vi "tipos.vi"() -> ()   [LabVIEW 2013]
panel:
  out "Boolean Indicator/Output":bool
  in  "Boolean Control/Input":bool
  in  "Stop Button":bool
  out "Double-precision, floating-point Indicator/Output":dbl
  in  "Byte unsigned integer 0 to 255  Control/Input":u8
  out "Horizontal Graduated Bar Indicator/Output":u8(slide) scale=0.0..100.0
  in  "Vertical Pointer Slide Input Control/Input":dbl(slide) scale=0.0..10.0
  out "Gauge Indicator/Output":dbl(knob) scale=0.0..10.0
  out "String Indicator/Output":string
  in  "String Control/Input":string
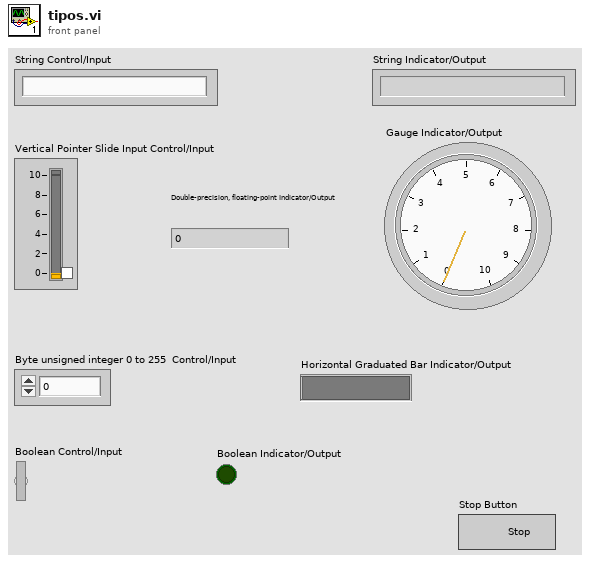
[diagram p1: front panel]
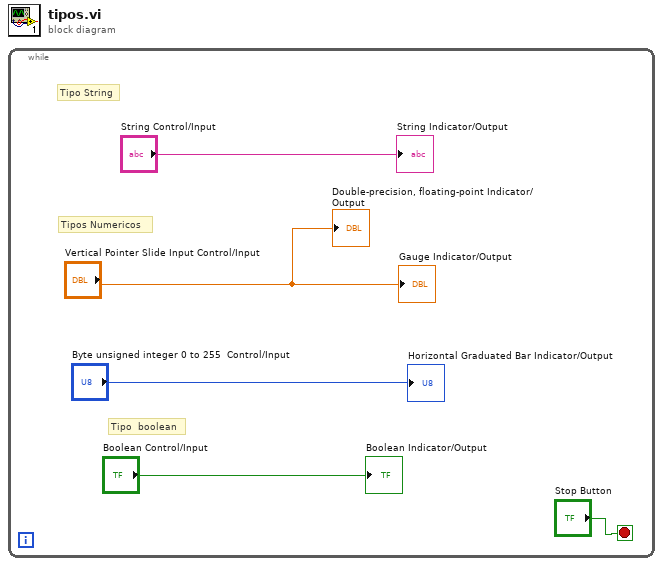
[diagram p0: block diagram]
diagram:
  n1 = while {
    stop <- "Stop Button" stop-if-true
    # "Tipo  boolean"
    # "Tipo String"
    # "Tipos Numericos"
    "String Indicator/Output" <- "String Control/Input"
    "Gauge Indicator/Output" <- "Vertical Pointer Slide Input Control/Input"
    "Horizontal Graduated Bar Indicator/Output" <- "Byte unsigned integer 0 to 255  Control/Input"
    "Double-precision, floating-point Indicator/Output" <- "Vertical Pointer Slide Input Control/Input"
    "Boolean Indicator/Output" <- "Boolean Control/Input"
  }
